vi "XML Reader Clone Handle.vi"(8 "error in (no error)":errorcluster, 11 "XML Reader In":T1) -> (0 "error out":errorcluster, 2 "XML Reader Copy":refnum<data-value>, 3 "XML Reader Out":T1)   [LabVIEW 2017, in "Pathloss XML Reader.lvlib"]
uses:
  Pathloss XML Reader.lvlib
  Controls/XML Reader Data.ctl
  Controls/XML Reader Data Ref.ctl
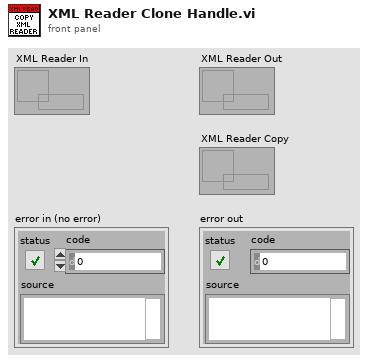
[diagram p1: front panel]
types:
  T1 = typedef "Pathloss XML Reader.lvlib/XML Reader Data Ref.ctl" = refnum<data-value>
  T2 = typedef "Pathloss XML Reader.lvlib/XML Reader Data.ctl" = cluster{"Remaining XML":string, "Section Name Stack":string[], "Section Stack":string[]}
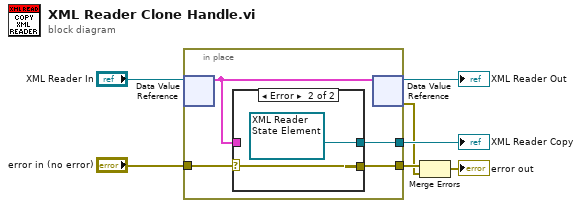
[diagram p0: block diagram]
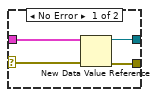
[diagram p2: hidden frame]
diagram:
  n1 = in-place {
    in-place-border: "error in (no error)" -> [w8]
    in-place-border: [w10] -> w3
    in-place-border: [w9] -> w2
    n2 = in-place-dvr #1("XML Reader In") -> (w11:T2)  [unwired: 1 out]
    n3 = case shown="Error" w8 {
      selector: w8 -> [w12 w16]
      tunnel: w11 -> [w15 _]
      tunnel: [w14 refnum<data-value> refnum ("data value reference")] -> w10
      tunnel: [w13 w16] -> w9
      frame No Error {
        n4 = New Data Value Reference(data value=w15, error in=w12) -> (data value reference=w14:refnum<data-value>, error out=w13:errorcluster)
      }
      frame Error {
      }
    }
    n5 = in-place-dvr #1(w11) -> (→"XML Reader Out":T1, w1:errorcluster)
  }
  "XML Reader Copy" <- w3
  n6 = Merge Errors(w2, w1) -> (→"error out":errorcluster)
